vi "Name (offset).vi"(8 "error in (no error)":errorcluster, 10 "offset (0)":i32, 11 "JSON":string) -> (0 "error out":errorcluster, 1 "JSON name":string, 2 "offset":i32)   [LabVIEW 2011, in "JSON Value.lvclass"]
doc: "Splits a JSON value string into a name and it's value. Unescapes the name.\n\nCopyright 2012 James David Powell, Shaun Rumbell and Ton Plomp\nMore information on http://lavag.org/topic/16217-cr-json-labview"
uses:
  JSON Value.lvclass
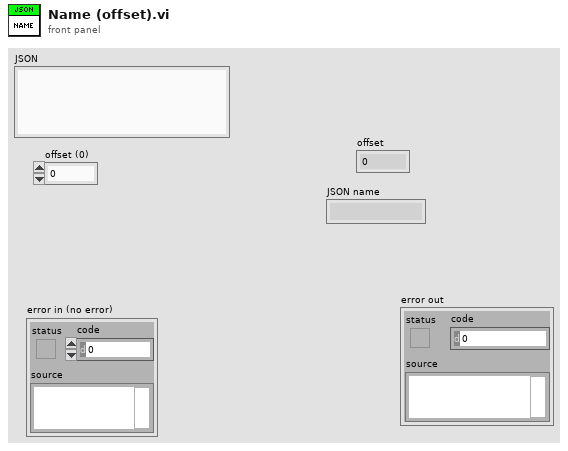
[diagram p1: front panel]
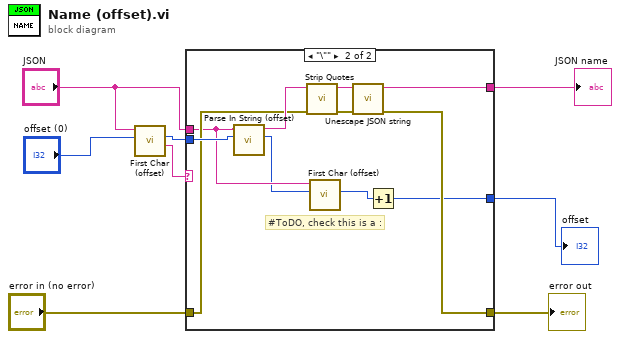
[diagram p0: block diagram]
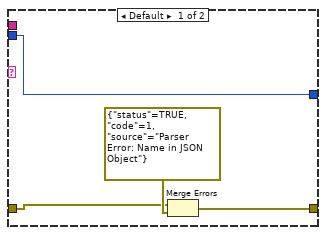
[diagram p2: hidden frame]
diagram:
  n1 = call "First Char (offset).vi"("offset (0)"="offset (0)", "String in"="JSON") -> ("First Char"=w5:string, "Offset"=w3:i32)  [unwired: 8 in]
  n2 = case shown="\"\\\"\"" w5 {
    tunnel: "JSON" -> [_ w14]
    tunnel: [_ w21] -> w8
    tunnel: [w10 w19] -> w7
    tunnel: "error in (no error)" -> [w11 w17]
    tunnel: w3 -> [w9 w18]
    tunnel: [w9 w15] -> w2
    frame Default {
      n3 = Merge Errors(w11, errorcluster {"status"=TRUE, "code"=1, "source"="Parser Error: Name in JSON Object"} ("error in")) -> (w10:errorcluster)
    }
    frame "\"" {
      # "#ToDO, check this is a :"
      n4 = call "Parse In String (offset).vi"("offset"=w18, "JSON (quote at offset)"=w14) -> ("offset"=w13:i32, "String (incl quotes)"=w23:string)  [unwired: 8 in]
      n5 = call "Strip Quotes.vi"("error in (no error)"=w17, "String"=w23) -> ("error out"=w20:errorcluster, "result string"=w22:string)  [unwired: 8 in]
      n6 = call "First Char (offset).vi"("offset (0)"=w13, "String in"=w14) -> ("Offset"=w16:i32)  [unwired: 8 in, 1 out]
      n7 = call "Unescape JSON string.vi"("error in (no error)"=w20, "Text (with JSON escapes)"=w22) -> ("error out"=w19:errorcluster, "Text (unescaped)"=w21:string)  [unwired: 8 in]
      n8 = Increment(x=w16) -> (x+1=w15:i32)
    }
  }
  "JSON name" <- w8
  "error out" <- w7
  "offset" <- w2
